vi "CustomDiagnostics.vi"() -> ()   [LabVIEW 2010]
uses:
  Status/CustomDiagPacketItem.ctl
panel:
  out "Axis Y DriveStatus all bits":dbl format="%#_6f"
  out "Axis X DriveStatus lowest 4 bits":dbl format="%#_6f"
  out "Task #1 TaskMode lowest 2 bits":dbl format="%#_6f"
  out "Global Double #4":dbl format="%#_6f"
  # "Custom Diagnostics is an advanced feature.\n\nPlease see the block diagram for the setup.\nThe items are retrieved all together, and\nthese items are the only one retrieved."
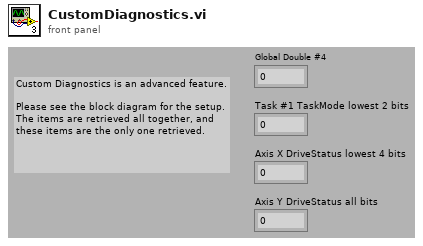
[diagram p1: front panel]
types:
  T1 = typedef "CustomDiagPacketItem.ctl" = cluster{"itemIndex":i16, "item code":u32, "extraArgument":i32}
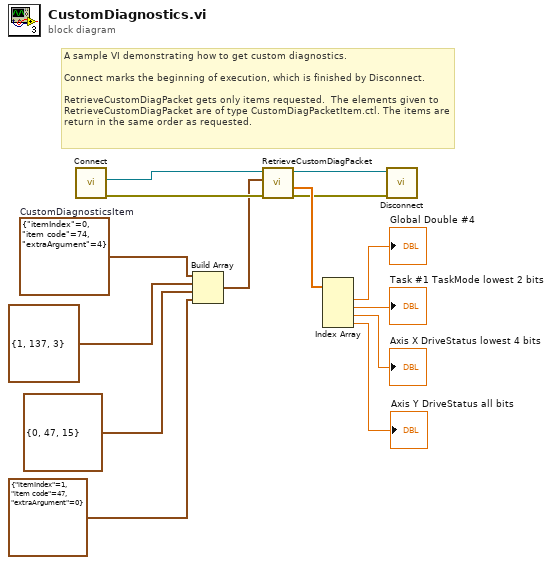
[diagram p0: block diagram]
diagram:
  w1 = T1 {"itemIndex"=0, "item code"=74, "extraArgument"=4}  # CustomDiagnosticsItem
  # "A sample VI demonstrating how to get custom diagnostics.\n\nConnect marks the beginning of execution, which is finished by Disconnect.\n\nRetrieveCustomDiagPacket gets only items requested.  The elements given to RetrieveCustomDiagPacket are of type CustomDiagPacketItem.ctl. The items are return in the same order as requested."
  n1 = call "Connect.vi"() -> ("error out"=w6:errorcluster, "controller"=w10:refnum<k24>)  [unwired: 10 in]
  n2 = Build Array(w1, T1 {"itemIndex"=1, "item code"=137, "extraArgument"=3} ("element"), T1 {"itemIndex"=0, "item code"=47, "extraArgument"=15} ("element"), T1 {"itemIndex"=1, "item code"=47, "extraArgument"=0} ("element")) -> (w5:T1[])
  n3 = call "RetrieveCustomDiagPacket.vi"("error in"=w6, "statusItems"=w5, "controller in"=w10) -> ("error out"=w7:errorcluster, "data"=w8:dbl[], "controller out"=w9:refnum<k24>)  [unwired: 6 in]
  n4 = Index Array(array=w8) -> (element #1=→"Global Double #4":dbl, element #2=→"Task #1 TaskMode lowest 2 bits":dbl, element #3=→"Axis X DriveStatus lowest 4 bits":dbl, element #4=→"Axis Y DriveStatus all bits":dbl)  [unwired: 4 in]
  n5 = call "Disconnect.vi"("error in (no error)"=w7, "controller"=w9) -> ()  [unwired: 9 in, 1 out]
